vi "Global Quit Event Holder.vi"() -> ()   [LabVIEW 2013, in "Template.lvlib" / "LQCoreEngine.lvclass"]
uses:
  LQCoreEngine.lvclass
panel:
  in  "Quit Event":refnum<user-event>
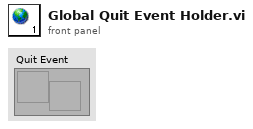
[diagram p1: front panel]
diagram:
